vi "Main.vi"() -> ()   [LabVIEW 2015]
uses:
  TypeDefs/Buttons UI.ctl
  TypeDefs/States.ctl
  TypeDefs/Acq Loop Data.ctl
panel:
  in  "#samples":dbl=100.0
  in  "Frequency":dbl=1000.0
  out "File Path":path
  in  "File Name Prefix":string="LV Academy"
  in  "Buttons":T1
  out "Wykres":dbl[](graph)
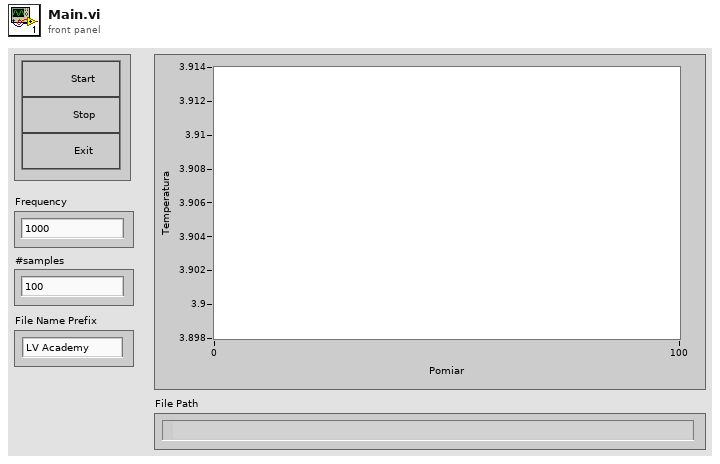
[diagram p1: front panel]
types:
  T1 = typedef "Buttons UI.ctl" = cluster{"Start":bool, "Stop":bool, "Exit":bool}
  T2 = typedef "Acq Loop Data.ctl" = cluster{"File Name Profix":string, "Frequency":dbl, "#samples":i32, "DAQ task ":refnum<k21>}
  T3 = typedef "Queue Data" = cluster{"Action":string, "Data":dbl[]}
  T4 = typedef "States.ctl" = enum16{"Check if Stop or Exit", "Exit", "Wait for Start or Exit", "Start Acquisition", "Reset Acquisition", "Acquisition"}
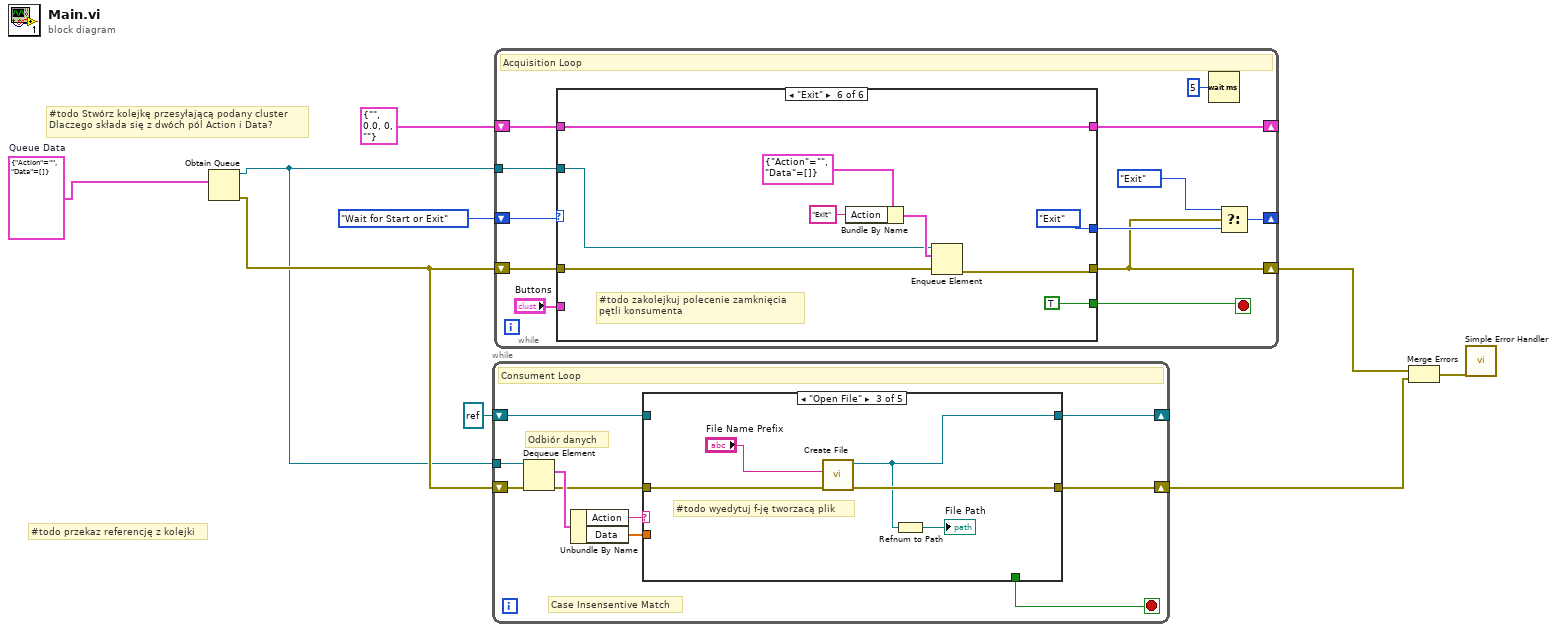
[diagram p0: block diagram]
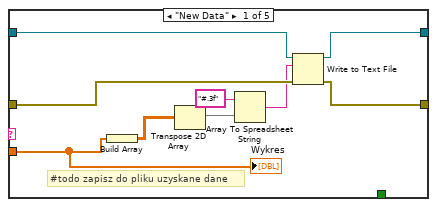
[diagram p2: hidden frame]
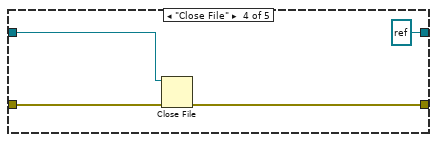
[diagram p4: hidden frame]
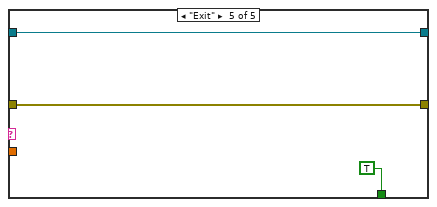
[diagram p5: hidden frame]
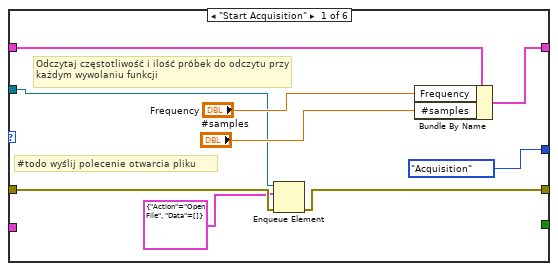
[diagram p6: hidden frame]
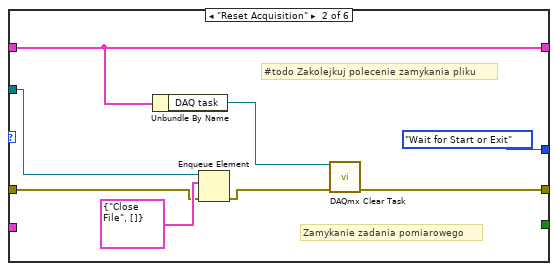
[diagram p7: hidden frame]
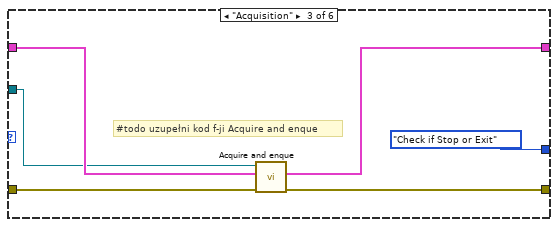
[diagram p8: hidden frame]
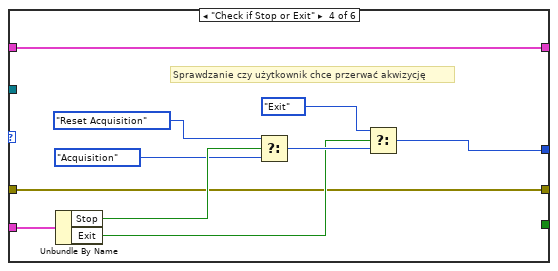
[diagram p9: hidden frame]
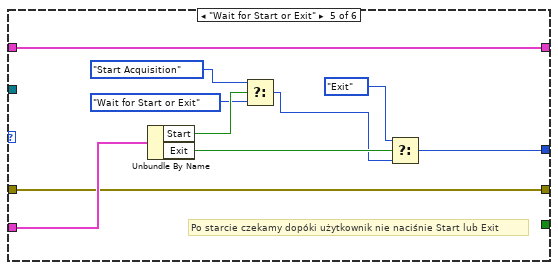
[diagram p10: hidden frame]
diagram:
  w3 = T3 {"Action"="", "Data"=[]}  # Queue Data
  # "#todo przekaz referencję z kolejki"
  # "#todo Stwórz kolejkę przesyłającą podany cluster\nDlaczego składa się z dwóch pól Action i Data?"
  n1 = Obtain Queue(element data type=w3) -> (queue out=w1:refnum<queue>, error out=w2:errorcluster)  [unwired: 4 in, 1 out]
  n2 = while {
    shift-right: [w13] -> w6
    shift-left: w2 -> [w19]
    shift-right: [w14] -> _
    shift-left: refnum<file> refnum ("refnum out") -> [w12]
    tunnel: w1 -> [w10]
    stop <- w11 stop-if-true
    # "Odbiór danych"
    # "Case Insensentive Match"
    # "Consument Loop"
    n3 = Dequeue Element(queue=w10, error in (no error)=w19) -> (element=w18:T3, error out=w15:errorcluster)  [unwired: 1 in, 2 out]
    n4 = Unbundle By Name(w18) -> ("Action"=w17:string, "Data"=w16:dbl[])
    n5 = case shown="\"Open File\"" w17 {
      tunnel: w16 -> [w28 _ _ _ _]
      tunnel: w15 -> [w23 w30 w35 w39 w41]
      tunnel: [w20 w29 w31 refnum<file> refnum ("refnum out") w40] -> w14
      tunnel: [w24 w30 w33 w37 w41] -> w13
      tunnel: w12 -> [w21 w29 _ w38 w40]
      tunnel: [_ _ _ _ TRUE] -> w11
      frame "New Data" {
        # "#todo zapisz do pliku uzyskane dane"
        n6 = Build Array(w28) -> (w27:dbl[][])
        n7 = Transpose 2D Array(2D array=w27) -> (transposed array=w26:dbl[][])
        n8 = Array To Spreadsheet String(array=w26, 3:"#.3f" ("format string")) -> (spreadsheet string=w22:string)  [unwired: 1 in]
        n9 = Write to Text File(file (use dialog)=w21, text=w22, error in=w23) -> (refnum out=w20:refnum<file>, error out=w24:errorcluster)  [unwired: 1 in, 1 out]
        "Wykres" <- w28
      }
      frame Default {
      }
      frame "Open File" {
        # "#todo wyedytuj f-ję tworzacą plik"
        n10 = call "Create File.vi"("error in (no error)"=w35, "File Name Prefix"="File Name Prefix") -> ("error out"=w33:errorcluster, "refnum out"=w31:refnum<file>)  [unwired: 8 in]
        n11 = Refnum to Path(1:w31) -> (0:→"File Path":path)
      }
      frame "Close File" {
        n12 = Close File(refnum=w38, error in=w39) -> (error out=w37:errorcluster)  [unwired: 1 out]
      }
      frame "Exit" {
      }
    }
  }
  n13 = while {
    shift-right: [w46] -> _
    shift-left: States."Wait for Start or Exit" -> [w54]
    shift-right: [w50] -> _
    shift-left: T2 {"File Name Profix"="", "Frequency"=0.0, "#samples"=0, "DAQ task "=""} -> [w51]
    shift-right: [w44] -> w5
    shift-left: w2 -> [w53]
    tunnel: w1 -> [w43]
    stop <- w48 stop-if-true
    # "Acquisition Loop"
    n14 = case shown="\"Exit\"" w54 {
      tunnel: w53 -> [w58 w65 w77 w79 w90 w99]
      tunnel: "Buttons" -> [_ _ _ w87 w97 _]
      tunnel: [States."Acquisition" States."Wait for Start or Exit" States."Check if Stop or Exit" w80 w92 States."Exit"] -> w47
      tunnel: w51 -> [w63 w68 w76 w78 w91 w103]
      tunnel: [w60 w68 w73 w78 w91 w103] -> w50
      tunnel: [w57 w71 w75 w79 w90 w98] -> w44
      tunnel: [_ _ _ _ _ TRUE] -> w48
      tunnel: w43 -> [w55 w66 w72 _ _ w100]
      frame "Start Acquisition" {
        # "#todo wyślij polecenie otwarcia pliku"
        # "Odczytaj częstotliwość i ilość próbek do odczytu przy każdym wywolaniu funkcji"
        n15 = Enqueue Element(queue=w55, element=T3 {"Action"="Open File", "Data"=[]}, error in (no error)=w58) -> (error out=w57:errorcluster)  [unwired: 1 in, 2 out]
        n16 = Bundle By Name(cluster=w63, "Frequency"="Frequency", "#samples"="#samples") -> (w60:T2)
      }
      frame "Reset Acquisition" {
        # "#todo Zakolejkuj polecenie zamykania pliku"
        # "Zamykanie zadania pomiarowego"
        n17 = Unbundle By Name(w68) -> ("DAQ task"=w70:refnum<k21>)
        n18 = Enqueue Element(queue=w66, element=T3 {"Action"="Close File", "Data"=[]}, error in (no error)=w65) -> (error out=w64:errorcluster)  [unwired: 1 in, 2 out]
        n19 = call <vilib>:"DAQmx Clear Task.vi"("task in"=w70, "error in"=w64) -> ("error out"=w71:errorcluster)  [unwired: 13 in]
      }
      frame "Acquisition" {
        # "#todo uzupełni kod f-ji Acquire and enque"
        n20 = call "Acquire and enque.vi"("error in (no error)"=w77, "Data In"=w76, "Queue in"=w72) -> ("error out"=w75:errorcluster, "Data Out"=w73:T2)  [unwired: 7 in]
      }
      frame "Check if Stop or Exit" {
        # "Sprawdzanie czy użytkownik chce przerwać akwizycję"
        n21 = Unbundle By Name(w87) -> ("Stop"=w86:bool, "Exit"=w82:bool)
        n22 = Select(t=States."Reset Acquisition", s=w86, f=States."Acquisition") -> (s? t:f=w83:T4)
        n23 = Select(t=States."Exit", s=w82, f=w83) -> (s? t:f=w80:T4)
      }
      frame "Wait for Start or Exit" {
        # "Po starcie czekamy dopóki użytkownik nie naciśnie Start lub Exit"
        n24 = Unbundle By Name(w97) -> ("Start"=w96:bool, "Exit"=w93:bool)
        n25 = Select(t=States."Start Acquisition", s=w96, f=States."Wait for Start or Exit") -> (s? t:f=w89:T4)
        n26 = Select(t=States."Exit", s=w93, f=w89) -> (s? t:f=w92:T4)
      }
      frame "Exit" {
        # "#todo zakolejkuj polecenie zamknięcia\npętli konsumenta"
        n27 = Bundle By Name(cluster=T3 {"Action"="", "Data"=[]}, "Action"="Exit") -> (w101:T3)
        n28 = Enqueue Element(queue=w100, element=w101, error in (no error)=w99) -> (error out=w98:errorcluster)  [unwired: 1 in, 2 out]
      }
    }
    n29 = Wait (ms)(milliseconds to wait=u32 5) -> ()  [unwired: 1 out]
    n30 = Select(t=States."Exit", s=w44, f=w47) -> (s? t:f=w46:T4)
  }
  n31 = Merge Errors(w5, w6) -> (w4:errorcluster)
  n32 = call <vilib>:"Simple Error Handler.vi"("error in (no error)"=w4) -> ()  [unwired: 4 in, 5 out]
